vi "FINAL.vi"() -> ()   [LabVIEW 2015]
uses:
  <vilib>/Instr/_visa.llb/VISA Configure Serial Port (Instr).vi
panel:
  out "AMARILLO 2":bool
  out "Thermometer":dbl(slide) scale=0.0..150.0
  out "Abastecimiento":dbl
  out "ROJO":bool
  out "VERDE":bool
  out "Tanque":dbl(slide) scale=0.0..2000.0
  out "Cisterna":dbl(slide) scale=0.0..40000.0
  in  "Llenar":bool
  in  "RESET":bool
  in  "Consumo u":bool
  in  "Consumo d":bool
  in  "CONSUMO":bool
  out "NIVEL 0":bool
  out "NIVEL 1":bool
  out "NIVEL 2":bool
  out "BA":bool
  out "B2":bool
  out "B1":bool
  out "NIVEL VACIO":bool
  in  "Litros para N0":dbl
  in  "Litros para N1":dbl
  in  "Litros para N2":dbl
  in  "Tanque":dbl
  in  "Temperatura":dbl
  in  "Consumo del tanque":dbl
  in  "Set Point mínimo":dbl
  in  "Set point máximo":dbl
  in  "BA":dbl
  in  "B1":dbl
  in  "B2":dbl
  in  "Litros en la cisterna":dbl
  in  "Nivel de vacío":dbl
  in  "temp down":bool
  in  "Temp up":bool
  in  "stop":bool
  in  "VISA resource name":refnum<visa-resource-name>
  # "TORRETA DE SEÑALIZACIÓN"
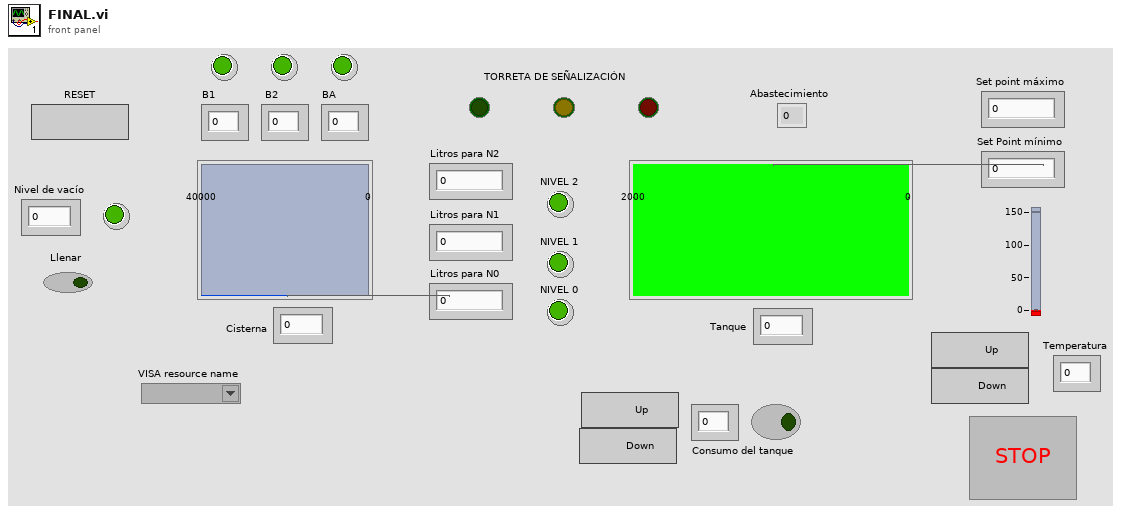
[diagram p1: front panel]
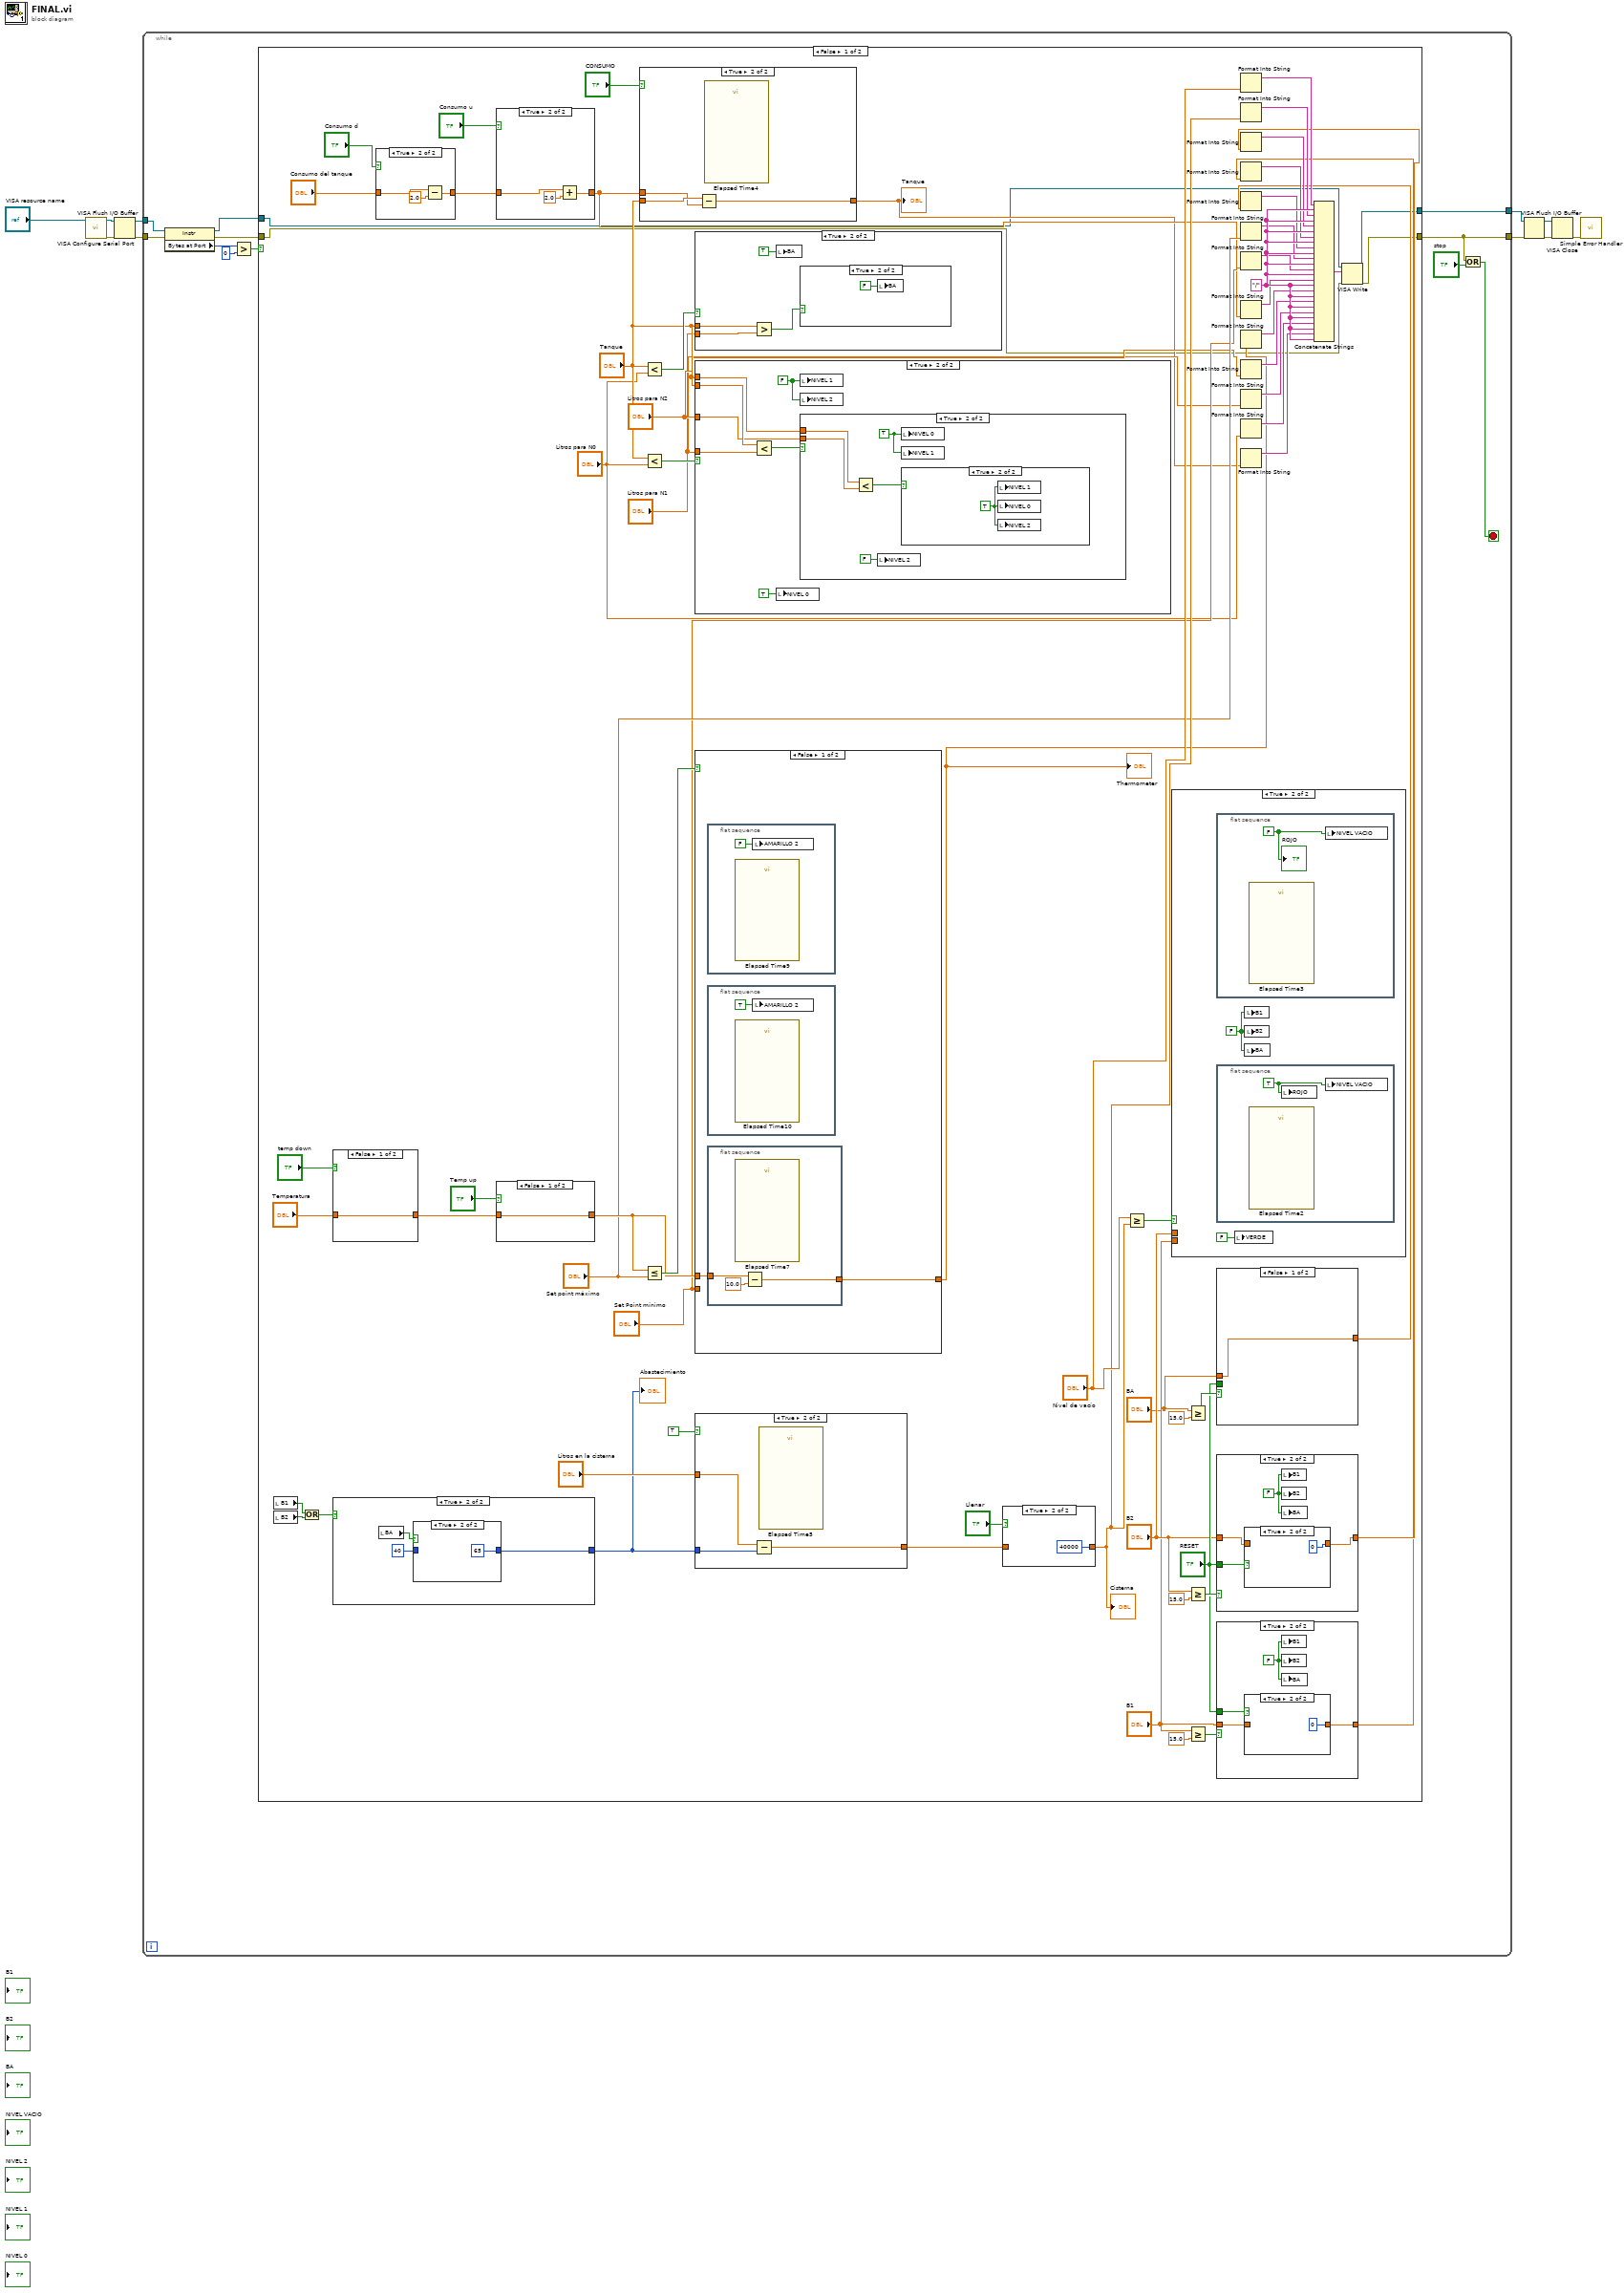
[diagram p0: block diagram]
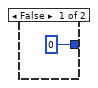
[diagram p3: hidden frame]
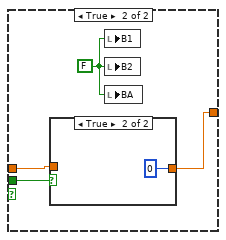
[diagram p9: hidden frame]
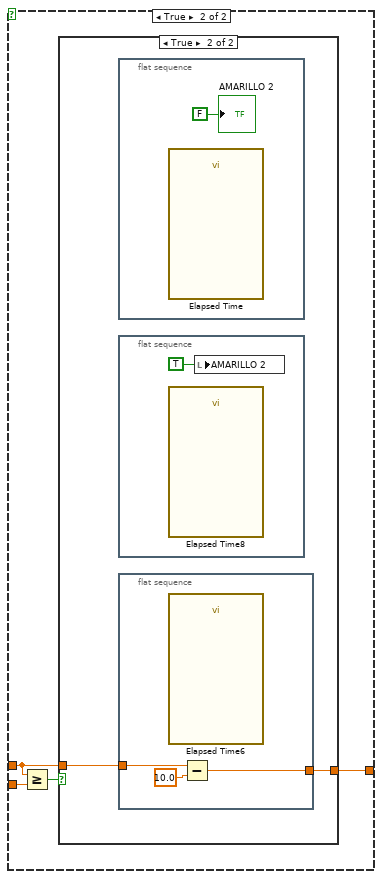
[diagram p18: hidden frame]
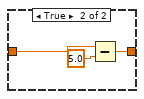
[diagram p20: hidden frame]
diagram:
  n1 = call-poly "VISA Configure Serial Port"("VISA resource name"="VISA resource name") -> ("VISA resource name out"=w10:refnum<visa-resource-name>, "error out"=w9:errorcluster)  [unwired: 13 in]
  n2 = VISA Flush I/O Buffer(VISA resource name=w10, error in (no error)=w9) -> (VISA resource name out=w7:refnum<visa-resource-name>, error out=w6:errorcluster)  [unwired: 1 in]
  n3 = while {
    tunnel: w7 -> [w19]
    tunnel: w6 -> [w18]
    tunnel: [w11] -> w1
    tunnel: [w12] -> w2
    stop <- w20 stop-if-true
    n4 = property class="Instr"(reference=w19, error in=w18) -> (reference out=w14:refnum<visa-resource-name>, error out=w17:errorcluster, "Bytes at Port"=w16:u32)
    n5 = Greater?(x=w16, y=u32 0) -> (0:w13:bool)
    n6 = case shown="False" w13 {
      tunnel: w17 -> [w22 w199]
      tunnel: [w24 w191] -> w11
      tunnel: w14 -> [w23 w200]
      tunnel: [w25 w192] -> w12
      frame False {
        w53 = "/"
        n7 = local read "B1"() -> (w60:bool)
        n8 = local read "B2"() -> (w59:bool)
        n9 = Or(x=w60, y=w59) -> (x .or. y?=w58:bool)
        n10 = case shown="False" "temp down" {
          tunnel: "Temperatura" -> [w164 w166]
          tunnel: [w164 w165] -> w82
          frame False {
          }
          frame True {
            n11 = Subtract(x=w166, y=5.0) -> (x-y=w165:dbl)
          }
        }
        n12 = case shown="True" w58 {
          tunnel: [0 w92] -> w54
          frame False {
          }
          frame True {
            n13 = local read "BA"() -> (w94:bool)
            n14 = case shown="True" w94 {
              tunnel: 40 -> [w95 _]
              tunnel: [w95 65] -> w92
              frame False {
              }
              frame True {
              }
            }
          }
        }
        "Abastecimiento" <- w54
        n15 = case shown="True" "Consumo d" {
          tunnel: "Consumo del tanque" -> [w133 w135]
          tunnel: [w133 w134] -> w77
          frame False {
          }
          frame True {
            n16 = Subtract(x=w135, y=2.0) -> (x-y=w134:dbl)
          }
        }
        n17 = case shown="True" "Consumo u" {
          tunnel: w77 -> [w137 w139]
          tunnel: [w137 w138] -> w32
          frame False {
          }
          frame True {
            n18 = Add(x=w139, y=2.0) -> (x+y=w138:dbl)
          }
        }
        n19 = case shown="False" "Temp up" {
          tunnel: w82 -> [w168 w170]
          tunnel: [w168 w169] -> w80
          frame False {
          }
          frame True {
            n20 = Add(x=w170, y=5.0) -> (x+y=w169:dbl)
          }
        }
        n21 = case shown="True" "CONSUMO" {
          tunnel: "Tanque" -> [w141 w144]
          tunnel: w32 -> [_ w143]
          tunnel: [w141 w142] -> w27
          frame False {
          }
          frame True {
            n22 = Subtract(x=w144, y=w143) -> (x-y=w142:dbl)
            n23 = call "Elapsed Time4"() -> ()  [unwired: 12 in, 8 out]
          }
        }
        "Tanque" <- w27
        n24 = Less?(x="Tanque", y="Litros para N0") -> (x < y?=w85:bool)
        n25 = Less?(x="Tanque", y="Litros para N0") -> (x < y?=w62:bool)
        n26 = Less Or Equal?(x=w80, y="Set point máximo") -> (x <= y?=w81:bool)
        n27 = case shown="True" w85 {
          tunnel: "Tanque" -> [_ w174]
          tunnel: "Litros para N1" -> [_ w173]
          frame False {
            n28 = local write "BA"(FALSE) -> ()
          }
          frame True {
            n29 = Greater?(x=w174, y=w173) -> (0:w175:bool)
            n30 = local write "BA"(TRUE) -> ()
            n31 = case shown="True" w175 {
              frame False {
              }
              frame True {
                n32 = local write "BA"(FALSE) -> ()
              }
            }
          }
        }
        n33 = case shown="True" w62 {
          tunnel: "Tanque" -> [_ w102]
          tunnel: "Tanque" -> [_ w101]
          tunnel: "Litros para N1" -> [_ w100]
          tunnel: "Litros para N2" -> [_ w99]
          frame False {
          }
          frame True {
            w97 = FALSE
            n34 = Less?(x=w102, y=w100) -> (x < y?=w103:bool)
            n35 = local write "NIVEL 0"(TRUE) -> ()
            n36 = local write "NIVEL 1"(w97) -> ()
            n37 = local write "NIVEL 2"(w97) -> ()
            n38 = case shown="True" w103 {
              tunnel: w101 -> [_ w107]
              tunnel: w99 -> [_ w106]
              frame False {
              }
              frame True {
                w105 = TRUE
                n39 = Less?(x=w107, y=w106) -> (x < y?=w108:bool)
                n40 = local write "NIVEL 2"(FALSE) -> ()
                n41 = local write "NIVEL 0"(w105) -> ()
                n42 = local write "NIVEL 1"(w105) -> ()
                n43 = case shown="True" w108 {
                  frame False {
                  }
                  frame True {
                    w109 = TRUE
                    n44 = local write "NIVEL 1"(w109) -> ()
                    n45 = local write "NIVEL 0"(w109) -> ()
                    n46 = local write "NIVEL 2"(w109) -> ()
                  }
                }
              }
            }
          }
        }
        n47 = case shown="False" w81 {
          tunnel: w80 -> [w146 w154]
          tunnel: [w145 w153] -> w31
          tunnel: "Set Point mínimo" -> [_ w155]
          frame False {
            n48 = flat-sequence {
              frame #0 {
                n49 = call "Elapsed Time9"() -> ()  [unwired: 12 in, 8 out]
                n50 = local write "AMARILLO 2"(FALSE) -> ()
              }
            }
            n51 = flat-sequence {
              frame #0 {
                n52 = call "Elapsed Time10"() -> ()  [unwired: 12 in, 8 out]
                n53 = local write "AMARILLO 2"(TRUE) -> ()
              }
            }
            n54 = flat-sequence {
              tunnel: w146 -> [w148]
              tunnel: [w147] -> w145
              frame #0 {
                n55 = call "Elapsed Time7"() -> ()  [unwired: 12 in, 8 out]
                n56 = Subtract(x=w148, y=10.0) -> (x-y=w147:dbl)
              }
            }
          }
          frame True {
            n57 = Greater Or Equal?(x=w154, y=w155) -> (x >= y?=w152:bool)
            n58 = case shown="True" w152 {
              tunnel: w154 -> [w156 w158]
              tunnel: [w156 w157] -> w153
              frame False {
              }
              frame True {
                n59 = flat-sequence {
                  frame #0 {
                    n60 = call "Elapsed Time"() -> ()  [unwired: 12 in, 8 out]
                    "AMARILLO 2" <- FALSE
                  }
                }
                n61 = flat-sequence {
                  frame #0 {
                    n62 = call "Elapsed Time8"() -> ()  [unwired: 12 in, 8 out]
                    n63 = local write "AMARILLO 2"(TRUE) -> ()
                  }
                }
                n64 = flat-sequence {
                  tunnel: w158 -> [w161]
                  tunnel: [w159] -> w157
                  frame #0 {
                    n65 = call "Elapsed Time6"() -> ()  [unwired: 12 in, 8 out]
                    n66 = Subtract(x=w161, y=10.0) -> (x-y=w159:dbl)
                  }
                }
              }
            }
          }
        }
        "Thermometer" <- w31
        n67 = case shown="True" TRUE {
          tunnel: w54 -> [_ w89]
          tunnel: "Litros en la cisterna" -> [w87 w90]
          tunnel: [w87 w88] -> w55
          frame False {
          }
          frame True {
            n68 = Subtract(x=w90, y=w89) -> (x-y=w88:dbl)
            n69 = call "Elapsed Time5"() -> ()  [unwired: 12 in, 8 out]
          }
        }
        n70 = case shown="True" "Llenar" {
          tunnel: w55 -> [w110 _]
          tunnel: [w110 40000] -> w38
          frame False {
          }
          frame True {
          }
        }
        "Cisterna" <- w38
        n71 = Greater Or Equal?(x="Nivel de vacío", y=w38) -> (x >= y?=w86:bool)
        n72 = case shown="True" w86 {
          tunnel: "B2" -> [w180 _]
          tunnel: "B1" -> [w179 _]
          frame False {
            n73 = Greater?(x=w180, y=w179) -> (0:w181:bool)
            n74 = local write "NIVEL VACIO"(FALSE) -> ()
            n75 = case shown="False" w181 {
              frame False {
                n76 = local write "B1"(TRUE) -> ()
                n77 = local write "B2"(FALSE) -> ()
              }
              frame True {
                n78 = local write "B1"(FALSE) -> ()
                n79 = local write "B2"(TRUE) -> ()
              }
            }
            "VERDE" <- TRUE
          }
          frame True {
            w188 = FALSE
            n80 = flat-sequence {
              frame #0 {
                w189 = FALSE
                n81 = call "Elapsed Time3"() -> ()  [unwired: 12 in, 8 out]
                n82 = local write "NIVEL VACIO"(w189) -> ()
                "ROJO" <- w189
              }
            }
            n83 = flat-sequence {
              frame #0 {
                w190 = TRUE
                n84 = call "Elapsed Time2"() -> ()  [unwired: 12 in, 8 out]
                n85 = local write "ROJO"(w190) -> ()
                n86 = local write "NIVEL VACIO"(w190) -> ()
              }
            }
            n87 = local write "VERDE"(FALSE) -> ()
            n88 = local write "B1"(w188) -> ()
            n89 = local write "B2"(w188) -> ()
            n90 = local write "BA"(w188) -> ()
          }
        }
        n91 = Greater Or Equal?(x="BA", y=15.0) -> (x >= y?=w68:bool)
        n92 = Greater Or Equal?(x="B2", y=15.0) -> (x >= y?=w72:bool)
        n93 = Greater Or Equal?(x="B1", y=15.0) -> (x >= y?=w71:bool)
        n94 = case shown="False" w68 {
          tunnel: "RESET" -> [_ w115]
          tunnel: "BA" -> [w112 w114]
          tunnel: [w112 w113] -> w35
          frame False {
          }
          frame True {
            w116 = FALSE
            n95 = case shown="True" w115 {
              tunnel: w114 -> [w117 _]
              tunnel: [w117 0] -> w113
              frame False {
              }
              frame True {
              }
            }
            n96 = local write "B1"(w116) -> ()
            n97 = local write "B2"(w116) -> ()
            n98 = local write "BA"(w116) -> ()
          }
        }
        n99 = case shown="True" w72 {
          tunnel: "RESET" -> [_ w129]
          tunnel: [w126 w127] -> w37
          tunnel: "B2" -> [w126 w128]
          frame False {
          }
          frame True {
            w130 = FALSE
            n100 = case shown="True" w129 {
              tunnel: w128 -> [w131 _]
              tunnel: [w131 0] -> w127
              frame False {
              }
              frame True {
              }
            }
            n101 = local write "B1"(w130) -> ()
            n102 = local write "B2"(w130) -> ()
            n103 = local write "BA"(w130) -> ()
          }
        }
        n104 = case shown="True" w71 {
          tunnel: "RESET" -> [_ w122]
          tunnel: [w119 w120] -> w36
          tunnel: "B1" -> [w119 w121]
          frame False {
          }
          frame True {
            w123 = FALSE
            n105 = case shown="True" w122 {
              tunnel: [w124 0] -> w120
              tunnel: w121 -> [w124 _]
              frame False {
              }
              frame True {
              }
            }
            n106 = local write "B1"(w123) -> ()
            n107 = local write "B2"(w123) -> ()
            n108 = local write "BA"(w123) -> ()
          }
        }
        n109 = Format Into String("Nivel de vacío") -> (resulting string=w52:string)  [unwired: 3 in, 1 out]
        n110 = Format Into String(w38) -> (resulting string=w51:string)  [unwired: 3 in, 1 out]
        n111 = Format Into String(w37) -> (resulting string=w50:string)  [unwired: 3 in, 1 out]
        n112 = Format Into String(w36) -> (resulting string=w49:string)  [unwired: 3 in, 1 out]
        n113 = Format Into String(w35) -> (resulting string=w48:string)  [unwired: 3 in, 1 out]
        n114 = Format Into String("Set point máximo") -> (resulting string=w47:string)  [unwired: 3 in, 1 out]
        n115 = Format Into String("Set Point mínimo") -> (resulting string=w46:string)  [unwired: 3 in, 1 out]
        n116 = Format Into String(w32) -> (resulting string=w45:string)  [unwired: 3 in, 1 out]
        n117 = Format Into String(w31) -> (resulting string=w44:string)  [unwired: 3 in, 1 out]
        n118 = Format Into String("Litros para N2") -> (resulting string=w43:string)  [unwired: 3 in, 1 out]
        n119 = Format Into String("Litros para N1") -> (resulting string=w42:string)  [unwired: 3 in, 1 out]
        n120 = Format Into String("Litros para N0") -> (resulting string=w41:string)  [unwired: 3 in, 1 out]
        n121 = Format Into String(w27) -> (resulting string=w40:string)  [unwired: 3 in, 1 out]
        n122 = Concatenate Strings(w52, w53, w51, w53, w50, w53, w49, w53, w48, w53, w47, w53, w46, w53, w45, w53, w44, w53, w43, w53, w42, w53, w41, w53, w40, w53) -> (w26:string)
        n123 = VISA Write(VISA resource name=w23, write buffer=w26, error in (no error)=w22) -> (VISA resource name out=w25:refnum<visa-resource-name>, error out=w24:errorcluster)  [unwired: 1 out]
      }
      frame True {
        n124 = VISA Read(VISA resource name=w200, byte count=u32 1, error in (no error)=w199) -> (VISA resource name out=w196:refnum<visa-resource-name>, read buffer=w195:string, error out=w197:errorcluster)  [unwired: 1 out]
        n125 = Equal?(x=w195, y="@") -> (x = y?=w193:bool)
        n126 = case shown="True" w193 {
          tunnel: w197 -> [w201 w252]
          tunnel: w196 -> [w202 w253]
          tunnel: [w202 w219] -> w192
          tunnel: [w201 w220] -> w191
          frame False {
          }
          frame True {
            n127 = VISA Read(VISA resource name=w253, byte count=u32 56, error in (no error)=w252) -> (VISA resource name out=w219:refnum<visa-resource-name>, read buffer=w245:string, error out=w220:errorcluster)  [unwired: 1 out]
            n128 = Match Pattern(string=w245, regular expression="/" ("read buffer")) -> (before substring=w249:string, after substring=w248:string)  [unwired: 1 in, 2 out]
            n129 = Decimal String To Number(string=w249) -> (number=w218:i32)  [unwired: 2 in, 1 out]
            n130 = Match Pattern(string=w248, regular expression="/") -> (before substring=w246:string, after substring=w236:string)  [unwired: 1 in, 2 out]
            n131 = local write "Nivel de vacío"(w218) -> ()
            n132 = Decimal String To Number(string=w246) -> (number=w217:i32)  [unwired: 2 in, 1 out]
            n133 = Match Pattern(string=w236, regular expression="/") -> (before substring=w243:string, after substring=w235:string)  [unwired: 1 in, 2 out]
            n134 = local write "Litros en la cisterna"(w217) -> ()
            n135 = Decimal String To Number(string=w243) -> (number=w216:i32)  [unwired: 2 in, 1 out]
            n136 = Match Pattern(string=w235, regular expression="/") -> (before substring=w241:string, after substring=w234:string)  [unwired: 1 in, 2 out]
            n137 = local write "B2"(w216) -> ()
            n138 = Decimal String To Number(string=w241) -> (number=w215:i32)  [unwired: 2 in, 1 out]
            n139 = Match Pattern(string=w234, regular expression="/") -> (before substring=w239:string, after substring=w233:string)  [unwired: 1 in, 2 out]
            n140 = local write "B1"(w215) -> ()
            n141 = Decimal String To Number(string=w239) -> (number=w214:i32)  [unwired: 2 in, 1 out]
            n142 = Match Pattern(string=w233, regular expression="/") -> (before substring=w237:string, after substring=w224:string)  [unwired: 1 in, 2 out]
            n143 = local write "BA"(w214) -> ()
            n144 = Decimal String To Number(string=w237) -> (number=w213:i32)  [unwired: 2 in, 1 out]
            n145 = Match Pattern(string=w224, regular expression="/") -> (before substring=w231:string, after substring=w223:string)  [unwired: 1 in, 2 out]
            n146 = local write "Set point máximo"(w213) -> ()
            n147 = Decimal String To Number(string=w231) -> (number=w212:i32)  [unwired: 2 in, 1 out]
            n148 = Match Pattern(string=w223, regular expression="/") -> (before substring=w229:string, after substring=w222:string)  [unwired: 1 in, 2 out]
            n149 = local write "Set Point mínimo"(w212) -> ()
            n150 = Decimal String To Number(string=w229) -> (number=w211:i32)  [unwired: 2 in, 1 out]
            n151 = Match Pattern(string=w222, regular expression="/") -> (before substring=w227:string, after substring=w221:string)  [unwired: 1 in, 2 out]
            n152 = local write "Consumo del tanque"(w211) -> ()
            n153 = Decimal String To Number(string=w227) -> (number=w210:i32)  [unwired: 2 in, 1 out]
            n154 = Match Pattern(string=w221, regular expression="/") -> (before substring=w226:string, after substring=w206:string)  [unwired: 1 in, 2 out]
            n155 = local write "Temperatura"(w210) -> ()
            n156 = Decimal String To Number(string=w226) -> (number=w209:i32)  [unwired: 2 in, 1 out]
            n157 = Match Pattern(string=w206, regular expression="/") -> (before substring=w205:string, after substring=w204:string)  [unwired: 1 in, 2 out]
            n158 = local write "Litros para N2"(w209) -> ()
            n159 = Decimal String To Number(string=w205) -> (number=w208:i32)  [unwired: 2 in, 1 out]
            n160 = Decimal String To Number(string=w204) -> (number=w207:i32)  [unwired: 2 in, 1 out]
            n161 = local write "Litros para N1"(w208) -> ()
            n162 = local write "Litros para N0"(w207) -> ()
          }
        }
      }
    }
    n163 = Or(x=w11, y="stop") -> (x .or. y?=w20:bool)
  }
  n164 = VISA Flush I/O Buffer(VISA resource name=w2, error in (no error)=w1) -> (VISA resource name out=w4:refnum<visa-resource-name>, error out=w3:errorcluster)  [unwired: 1 in]
  n165 = VISA Close(VISA resource name=w4, error in (no error)=w3) -> (error out=w5:errorcluster)
  n166 = call <vilib>:"Simple Error Handler.vi"("error in (no error)"=w5) -> ()  [unwired: 4 in, 5 out]
